vi "Initialize_Piezo_Stage_LAN.vi"(1 "error in":errorcluster, 2 "Host address/name":string) -> (0 "error out":errorcluster)   [LabVIEW 2009]
panel:
  out "All conn. axes":string[](array[string])
  out "TCP/IP settings out":T1={"Host address/name"="localhost", "Port"=50000, "Board"=0}
  in  "Interface":u16(ring)=1 items=["RS232", "TCP/IP", "USB"]
  in  "System no.":i32=1 min=1 max=4 step=1
  in  "TCP/IP settings":T2={"Host address/name"="141.84.139.199", "Port"=50000, "Board"=0, "TCP/IP Search?"=FALSE}
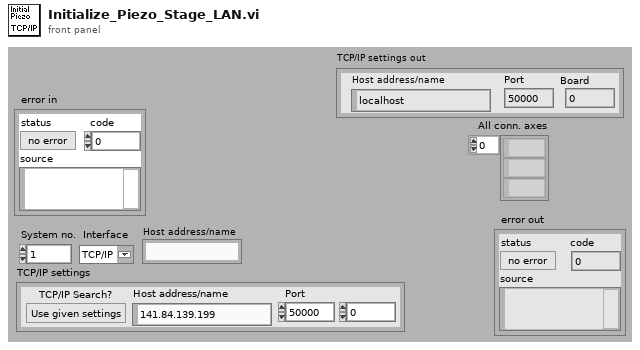
[diagram p1: front panel]
types:
  T1 = cluster{"Host address/name":string, "Port":i32, "Board":i32}
  T2 = cluster{"Host address/name":string, "Port":i32, "Board":i32, "TCP/IP Search?":bool}
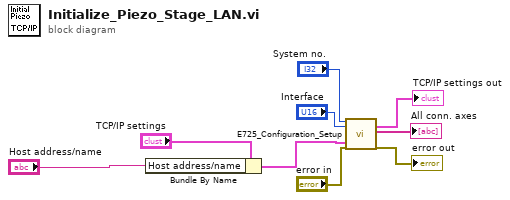
[diagram p0: block diagram]
diagram:
  n1 = Bundle By Name(cluster="TCP/IP settings", "Host address/name"="Host address/name") -> (w1:T2)
  n2 = call "E725_Configuration_Setup.vi"("System no."="System no.", "error in"="error in", "Interface"="Interface", "TCP/IP settings"=w1) -> ("TCP/IP settings out"=→"TCP/IP settings out":T1, "All conn. axes"=→"All conn. axes":string[], "error out"=→"error out":errorcluster)  [unwired: 11 in, 2 out]
